vi "Close MeasurementLink Session.vi"(8 "error in":errorcluster, 9 "initialize and close session behavior":T1, 10 "session in":variant, 11 "session factory in":refnum<class "Keysight_34401A-DMM.lvclass">) -> (0 "error out":errorcluster)   [LabVIEW 2020, in "Keysight_34401A-DMM.lvclass"]
doc: "Closes the local session. If the session represents a remote session, <b>initialize and close session behavior</b> determines whether closing the local session closes the server session or detaches from the server session."
uses:
  Keysight_34401A-DMM.lvclass
  <vilib>/MeasurementLink/MeasurementLink Instrument/ISession Factory/Initialize and Close Session Behavior.ctl
  Keysight_34401A-DMM.lvclass/Keysight_34401A-DMM.ctl
  <instrlib>/Agilent 34401/Public/Close.vi
  <instrlib>/Agilent 34401/Agilent 34401.lvlib
  <vilib>/MeasurementLink/MeasurementLink Instrument/ISession Factory/ISession Factory.lvclass
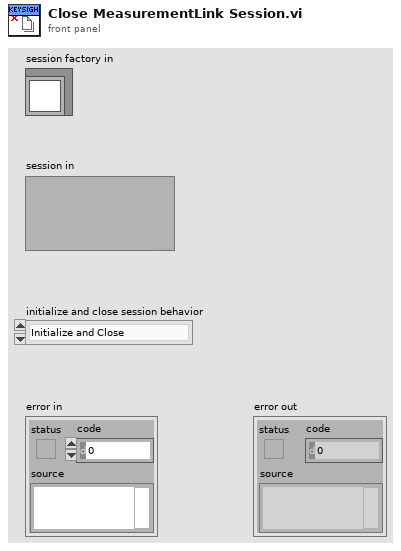
[diagram p1: front panel]
types:
  T1 = typedef "MeasurementLink Instrument.lvlib/ISession Factory.lvclass/Initialize and Close Session Behavior.ctl" = enum16{"Initialize and Close", "Attach and Detach", "Initialize and Detach", "Attach and Close"}
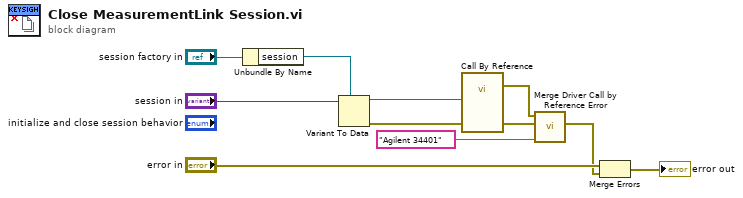
[diagram p0: block diagram]
diagram:
  n1 = Unbundle By Name("session factory in") -> ("session"=w1:refnum<visa-resource-name>)
  n2 = Variant To Data(type=w1, Variant="session in") -> (data=w6:refnum<visa-resource-name>, error out=w7:errorcluster)  [unwired: 1 in]
  n3 = call-by-ref "?"("error in (no error)"=w7, "VISA resource name"=w6) -> (error out=w9:errorcluster, 0:"error out"=w8:errorcluster)  [unwired: 11 in, 1 out]
  n4 = call <vilib>:"Merge Driver Call by Reference Error.vi"("driver name"="Agilent 34401", "called vi error"=w8, "call by ref error"=w9) -> ("error out"=w4:errorcluster)  [unwired: 8 in]
  n5 = Merge Errors("error in", w4) -> (→"error out":errorcluster)
